vi "Mux.vi"(0 "a":bool, 4 "sel":bool, 5 "b":bool) -> (7 "out":bool)   [LabVIEW 2014]
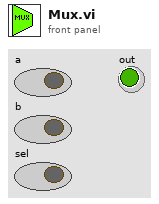
[diagram p1: front panel]
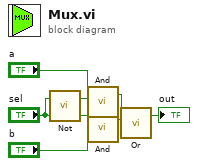
[diagram p0: block diagram]
diagram:
  n1 = call "Not.vi"("in"="sel") -> ("out"=w7:bool)  [unwired: 2 in]
  n2 = call "And.vi"("b"=w7, "a"="a") -> ("out"=w3:bool)  [unwired: 3 in]
  n3 = call "And.vi"("b"="b", "a"="sel") -> ("out"=w2:bool)  [unwired: 3 in]
  n4 = call "Or.vi"("b"=w2, "a"=w3) -> ("out"=→"out":bool)  [unwired: 3 in]
